vi "Low Limit is null.vi"(8 "error in":errorcluster, 11 "Object Entry in":refnum<class "Object Entry.lvclass">) -> (0 "error out":errorcluster, 2 "Null":bool=TRUE, 3 "Object Entry out":refnum<class "Object Entry.lvclass">)   [LabVIEW 2020, in "CANopen.lvlib" / "Object Entry.lvclass"]
uses:
  Object Entry.lvclass
  Object Entry.lvclass/Object Entry.ctl
  Sub Object/Sub Object.lvclass
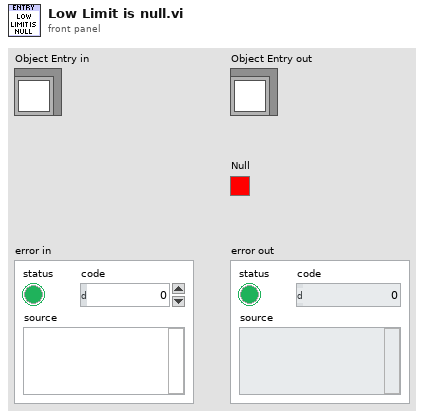
[diagram p1: front panel]
types:
  T1 = typedef "CANopen.lvlib/Object Type.ctl" = u8
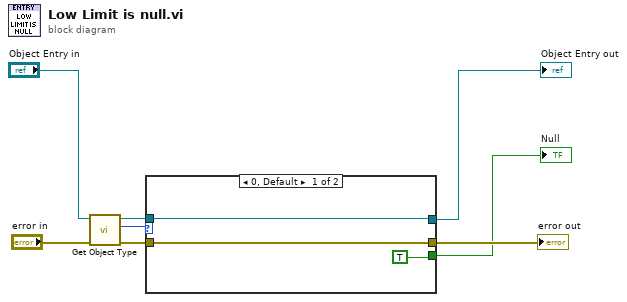
[diagram p0: block diagram]
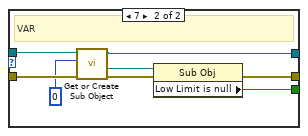
[diagram p2: hidden frame]
diagram:
  n1 = call "Get Object Type.vi"("error in"="error in", "Object Entry in"="Object Entry in") -> ("error out"=w7:errorcluster, "Object Type"=w4:T1, "Object Entry out"=w3:refnum<class "Object Entry.lvclass">)  [unwired: 7 in]
  n2 = case shown="0, Default" w4 {
    tunnel: w7 -> [w11 w19]
    tunnel: [w11 w18] -> w5
    tunnel: w3 -> [w9 w15]
    tunnel: [w9 w13] -> w2
    tunnel: [TRUE ("Low Limit is null") w12] -> w1
    frame 0, Default {
    }
    frame 7 {
      # "VAR"
      n3 = call "Get or Create Sub Object.vi"("error in"=w19, "Sub Index"=u8 0, "Obj Entry in"=w15) -> ("error out"=w17:errorcluster, "Sub Object"=w14:refnum<class "Sub Object.lvclass">, "Obj Entry out"=w13:refnum<class "Object Entry.lvclass">)  [unwired: 6 in]
      n4 = property class="Sub Obj"(reference=w14, error in=w17) -> (error out=w18:errorcluster, "Low Limit is null"=w12:bool)  [unwired: 1 out]
    }
  }
  "error out" <- w5
  "Object Entry out" <- w2
  "Null" <- w1
